vi "Create Serial Number File.vi"(8 "Error In":errorcluster) -> (0 "Error Out":errorcluster, 2 "Hardware Table":string[][](array[string]))   [LabVIEW 2010]
uses:
  <vilib>/Utility/file.llb/Write To Spreadsheet File (string).vi
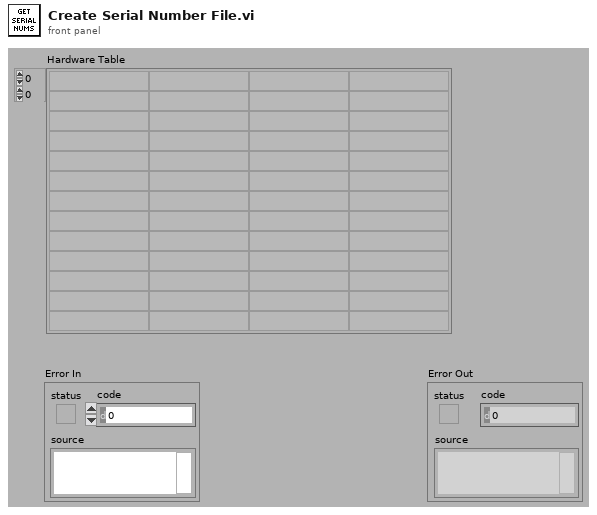
[diagram p1: front panel]
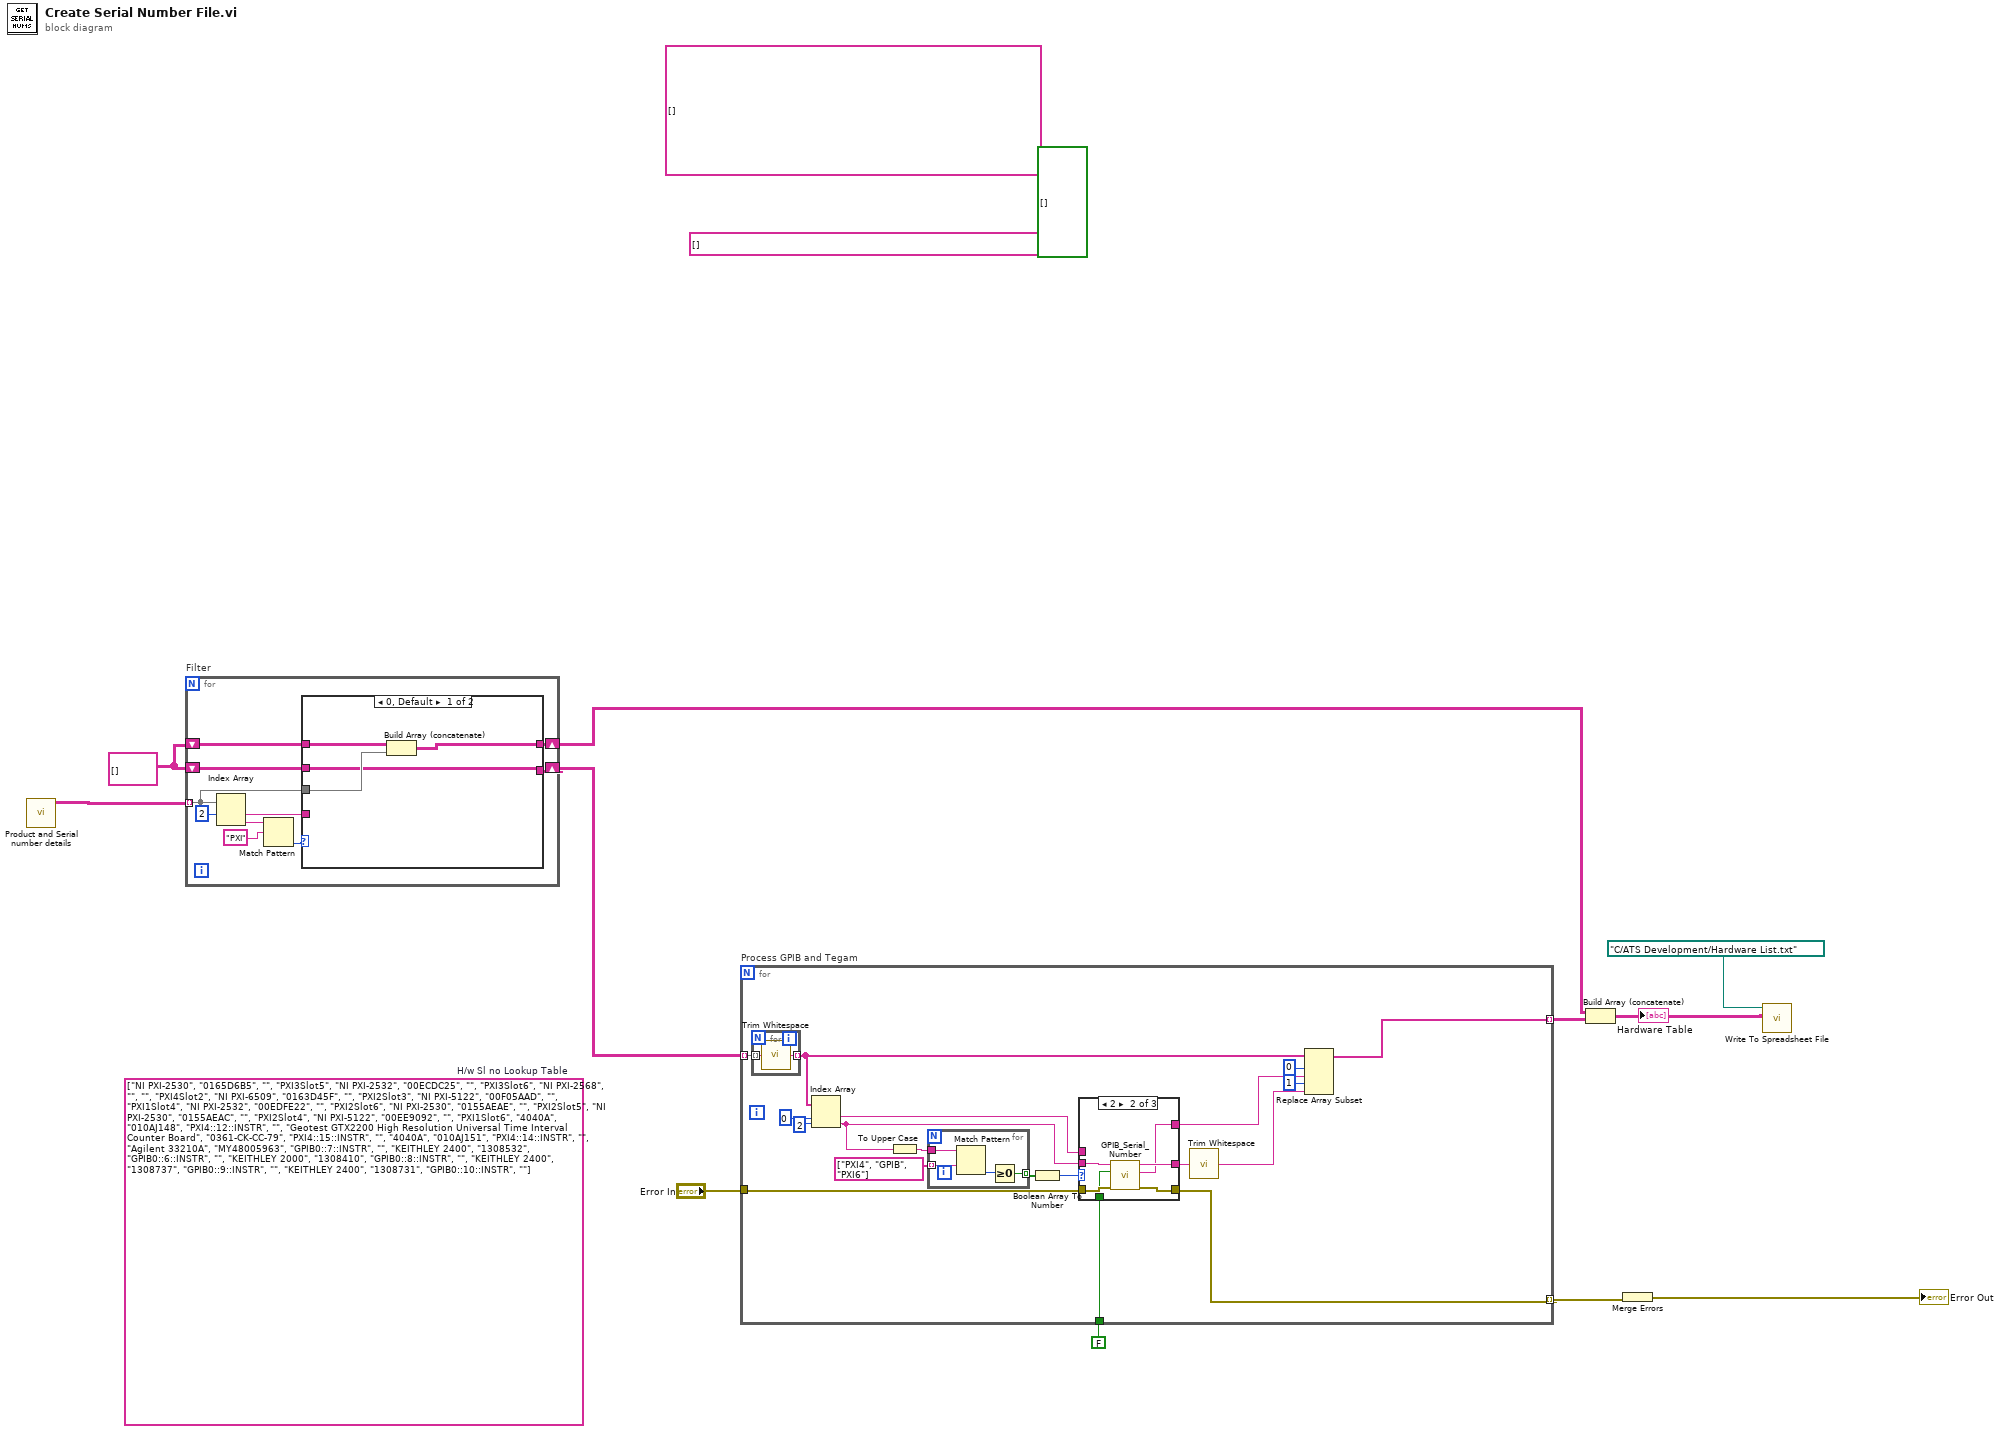
[diagram p0: block diagram]
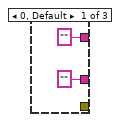
[diagram p2: hidden frame]
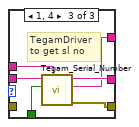
[diagram p3: hidden frame]
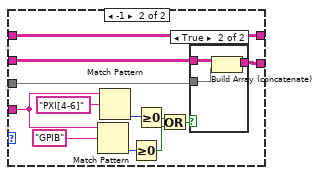
[diagram p4: hidden frame]
diagram:
  w10 = string[][] [] ("Lookup Table")
  (unwired) string[] []
  (unwired) string[][] []
  (unwired) bool[] []
  (unwired) string[][] [["NI PXI-2530", "0165D6B5", "", "PXI3Slot5"], ["NI PXI-2532", "00ECDC25", "", "PXI3Slot6"], ["NI PXI-2568", "", "", "PXI4Slot2"], ["NI PXI-6509", "0163D45F", "", "PXI2Slot3"], ["NI PXI-5122", "00F05AAD", "", "PXI1Slot4"], ["NI PXI-2532", "00EDFE22", "", "PXI2Slot6"], ["NI PXI-2530", "0155AEAE", "", "PXI2Slot5"], ["NI PXI-2530", "0155AEAC", "", "PXI2Slot4"], ["NI PXI-5122", "00EE9092", "", "PXI1Slot6"], ["4040A", "010AJ148", "PXI4::12::INSTR", ""], ["Geotest GTX2200 High Resolution Universal Time Interval Counter Board", "0361-CK-CC-79", "PXI4::15::INSTR", ""], ["4040A", "010AJ151", "PXI4::14::INSTR", ""], ["Agilent 33210A", "MY48005963", "GPIB0::7::INSTR", ""], ["KEITHLEY 2400", "1308532", "GPIB0::6::INSTR", ""], ["KEITHLEY 2000", "1308410", "GPIB0::8::INSTR", ""], ["KEITHLEY 2400", "1308737", "GPIB0::9::INSTR", ""], ["KEITHLEY 2400", "1308731", "GPIB0::10::INSTR", ""]]  # H/w Sl no Lookup Table
  n1 = call "Product and Serial number details.vi"() -> ("Product and Serial Number"=w9:string[][])  [unwired: 10 in, 1 out]
  n2 = for "Filter" {
    tunnel: w9 -> [w15] mode=indexing
    shift-right: [w14] -> w8
    shift-left: w10 -> [w16]
    shift-right: [w12] -> w4
    shift-left: w10 -> [w13]
    n3 = Index Array(array=w15, index #1=2 ("index")) -> (element #1=w17:string, element #2=w20:string)  [unwired: 1 in]
    n4 = Match Pattern(string=w20, regular expression="PXI") -> (offset past match=w18:i32)  [unwired: 1 in, 3 out]
    n5 = case shown="0, Default" w18 {
      tunnel: w17 -> [_ w35]
      tunnel: w16 -> [w22 w29]
      tunnel: w15 -> [w25 w28]
      tunnel: [w22 w27] -> w14
      tunnel: w13 -> [w24 w26]
      tunnel: [w23 w26] -> w12
      frame 0, Default {
        n6 = Build Array (concatenate)(w24, w25) -> (w23:string[][])
      }
      frame -1 {
        n7 = Match Pattern(string=w35, regular expression="GPIB") -> (offset past match=w33:i32)  [unwired: 1 in, 3 out]
        n8 = Match Pattern(string=w35, regular expression="PXI[4-6]") -> (offset past match=w34:i32)  [unwired: 1 in, 3 out]
        n9 = Greater Or Equal To 0?(x=w33) -> (x >= 0?=w32:bool)
        n10 = Greater Or Equal To 0?(x=w34) -> (x >= 0?=w31:bool)
        n11 = Or(x=w31, y=w32) -> (x .or. y?=w30:bool)
        n12 = case shown="True" w30 {
          tunnel: w29 -> [w38 w41]
          tunnel: w28 -> [_ w40]
          tunnel: [w38 w39] -> w27
          frame False {
          }
          frame True {
            n13 = Build Array (concatenate)(w41, w40) -> (w39:string[][])
          }
        }
      }
    }
  }
  n14 = for "Process GPIB and Tegam" {
    tunnel: w8 -> [w52] mode=indexing
    tunnel: "Error In" -> [w56]
    tunnel: [w54] -> w6 mode=indexing
    tunnel: FALSE -> [w53]
    tunnel: [w42] -> w3 mode=indexing
    n15 = for {
      tunnel: w52 -> [w62] mode=indexing
      tunnel: [w61] -> w47 mode=indexing
      n16 = call <vilib>:"Trim Whitespace.vi"("string"=w62) -> ("trimmed string"=w61:string)  [unwired: 1 in]
    }
    n17 = Index Array(array=w47, index #1=0 ("index"), index #2=2 ("index")) -> (element #1=w48:string, element #2=w49:string)
    n18 = To Upper Case(1:w49) -> (0:w60:string)
    n19 = for {
      tunnel: w60 -> [w80]
      tunnel: string[] ["PXI4", "GPIB", "PXI6"] -> [w79] mode=indexing
      tunnel: [w77] -> w58 mode=indexing
      n20 = Match Pattern(string=w80, regular expression=w79) -> (offset past match=w78:i32)  [unwired: 1 in, 3 out]
      n21 = Greater Or Equal To 0?(x=w78) -> (x >= 0?=w77:bool)
    }
    n22 = Boolean Array To Number(Boolean array=w58) -> (number=w57:u32)
    n23 = case shown="2" w57 {
      tunnel: ["" ("Serial Number") w67 w75] -> w55
      tunnel: w49 -> [_ w69 w73]
      tunnel: [_ w70 w76] -> w54
      tunnel: w56 -> [_ w68 _]
      tunnel: ["" ("Model") w66 w74] -> w46
      tunnel: w53 -> [_ w65 w72]
      tunnel: w48 -> [_ _ w71]
      frame 0, Default {
      }
      frame 2 {
        n24 = call "GPIB_Serial_Number.vi"("Error In"=w68, "Simulation"=w65, "GPIB Address"=w69) -> ("Error Out"=w70:errorcluster, "Model"=w66:string, "Serial Number"=w67:string)  [unwired: 6 in]
      }
      frame 1, 4 {
        # "TegamDriver\nto get sl no"
        n25 = call "Tegam_Serial_Number.vi"("Expected Model"=w71, "Simulation"=w72, "GPIB Address"=w73) -> ("Error Out"=w76:errorcluster, "Model"=w74:string, "Serial Number"=w75:string)  [unwired: 6 in]
      }
    }
    n26 = call <vilib>:"Trim Whitespace.vi"("string"=w55) -> ("trimmed string"=w45:string)  [unwired: 1 in]
    n27 = Replace Array Subset(array=w47, new element #1=w46, index #1=0 ("index"), new element #2=w45, index #2=1 ("index")) -> (w42:string[])
  }
  n28 = Build Array (concatenate)(w4, w3) -> (w2:string[][])
  "Hardware Table" <- w2
  n29 = Merge Errors(w6) -> (→"Error Out":errorcluster)
  n30 = call-poly <vilib>:"Write To Spreadsheet File.vi"("2D data"=w2, "file path (dialog if empty)"=path "C:/ATS Development/Hardware List.txt") -> ()  [unwired: 6 in, 1 out]
